vi "FindDevices.vi"(0 "Коммутатор Agilent 34980A":refnum<visa-resource-name>, 1 "Reset (True)":bool=TRUE, 5 "Мультиметр Agilent 34410A":refnum<visa-resource-name>, 7 "TP04300A":refnum<visa-resource-name>, 9 "Источник питания Agilent N6705A":refnum<visa-resource-name>) -> (4 "Статус коммутатора":bool, 6 "Статус вольтметра":bool, 8 "Статус камеры тепла/холода":bool, 10 "Статус источника питания":bool, 15 "error out":errorcluster)   [LabVIEW 2017]
uses:
  instr.lib/Temptronic TP04300/Temptronic TP04300.lvlib
  instr.lib/Agilent N6700 Series/Agilent N6700 Series.lvlib
panel:
  # "IN"
  # "OUT"
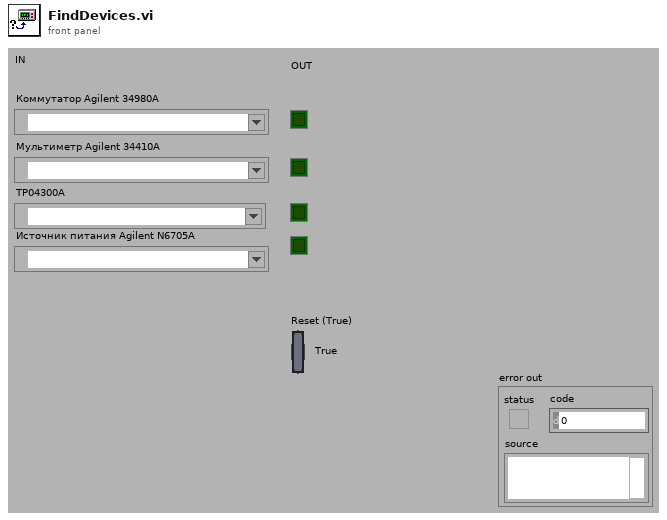
[diagram p1: front panel]
types:
  T1 = cluster{"Baud Rate":u32, "Parity":u16, "Data Bits":u16, "Stop Bits":u16, "Flow Control":u16}
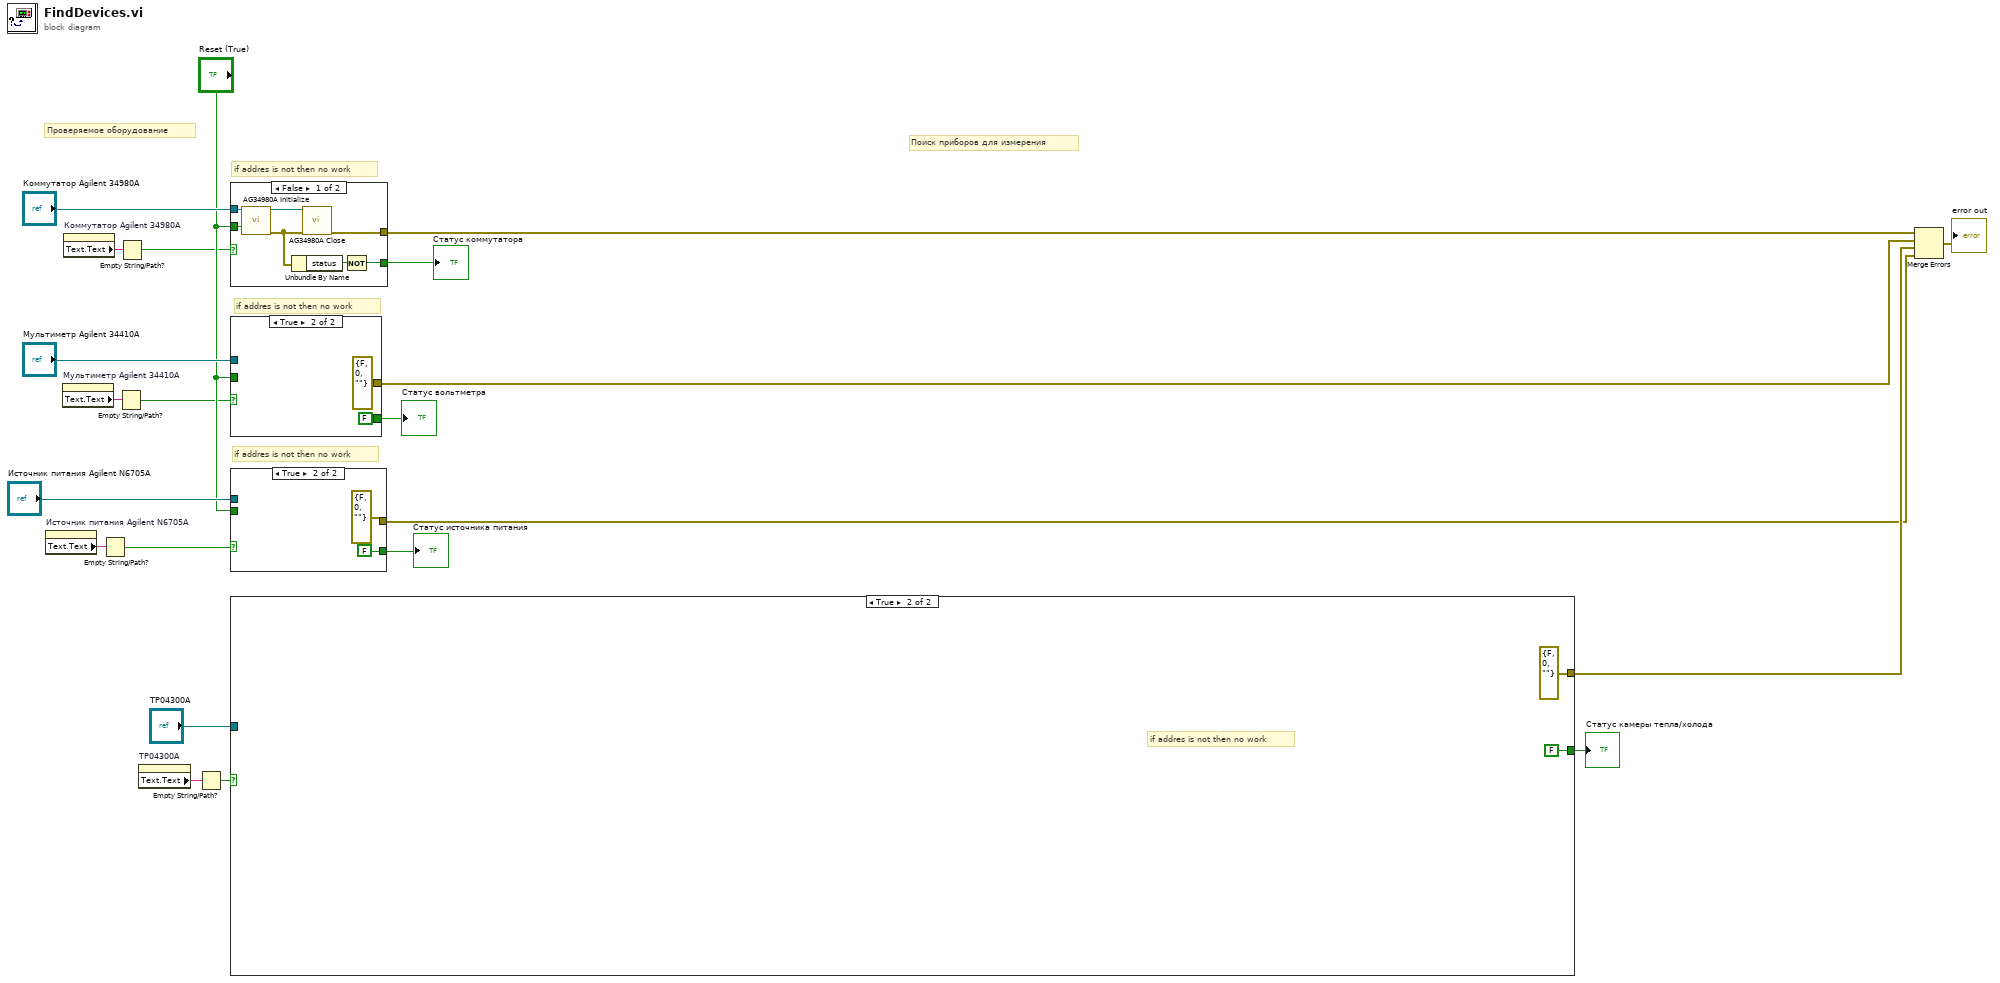
[diagram p0: block diagram]
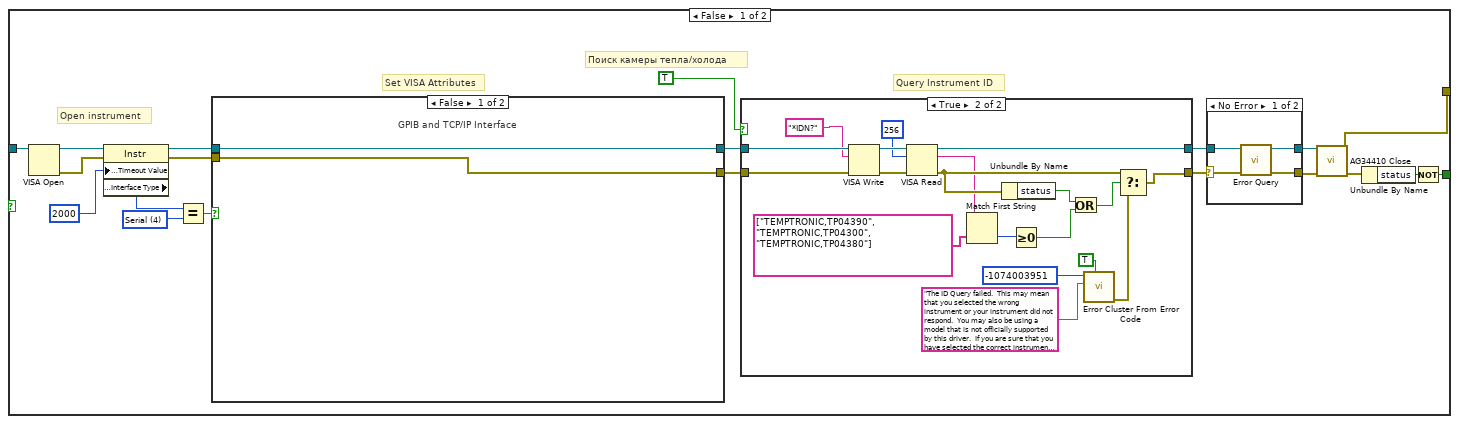
[diagram p2: hidden frame]
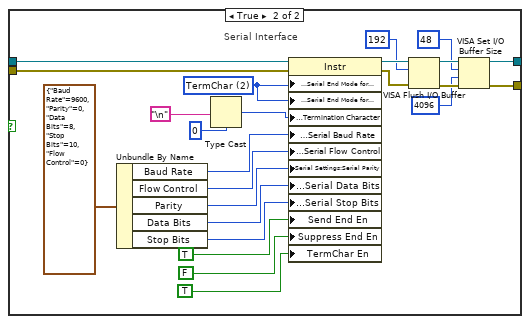
[diagram p3: hidden frame]
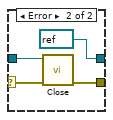
[diagram p4: hidden frame]
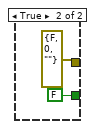
[diagram p6: hidden frame]
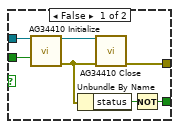
[diagram p7: hidden frame]
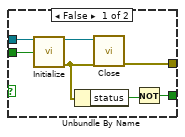
[diagram p8: hidden frame]
diagram:
  # "if addres is not then no work"
  # "if addres is not then no work"
  # "if addres is not then no work"
  # "if addres is not then no work"
  # "Проверяемое оборудование"
  # "Поиск приборов для измерения"
  n1 = property on="Источник питания Agilent N6705A" class="VISAName"() -> ("Text.Text"=w9:string)  [unwired: 2 in, 2 out]
  n2 = property on="Мультиметр Agilent 34410A" class="VISAName"() -> ("Text.Text"=w7:string)  [unwired: 2 in, 2 out]
  n3 = property on="Коммутатор Agilent 34980A" class="VISAName"() -> ("Text.Text"=w4:string)  [unwired: 2 in, 2 out]
  n4 = Empty String/Path?(string/path=w9) -> (empty?=w8:bool)
  n5 = Empty String/Path?(string/path=w7) -> (empty?=w6:bool)
  n6 = Empty String/Path?(string/path=w4) -> (empty?=w3:bool)
  n7 = property on="TP04300A" class="VISAName"() -> ("Text.Text"=w2:string)  [unwired: 2 in, 2 out]
  n8 = Empty String/Path?(string/path=w2) -> (empty?=w1:bool)
  n9 = case shown="False" w3 {
    tunnel: [w29 errorcluster {"status"=FALSE, "code"=0, "source"=""} ("error out")] -> w18
    tunnel: [w28 FALSE] -> w17
    tunnel: "Коммутатор Agilent 34980A" -> [w26 _]
    tunnel: "Reset (True)" -> [w23 _]
    frame False {
      n10 = call "AG34980A Initialize.vi"("VISA resource name"=w26, "Reset (True)"=w23) -> ("VISA session"=w25:refnum<visa-resource-name>, "error out"=w24:errorcluster)  [unwired: 12 in]
      n11 = Unbundle By Name(w24) -> ("status"=w27:bool)
      n12 = call "AG34980A Close.vi"("VISA resource name"=w25, "error in (no error)"=w24) -> ("error out"=w29:errorcluster)  [unwired: 13 in]
      n13 = Not(x=w27) -> (.not. x?=w28:bool)
    }
    frame True {
    }
  }
  "Статус коммутатора" <- w17
  n14 = case shown="True" w6 {
    tunnel: [w38 errorcluster {"status"=FALSE, "code"=0, "source"=""} ("error out")] -> w19
    tunnel: [w32 FALSE ("status")] -> w5
    tunnel: "Мультиметр Agilent 34410A" -> [w37 _]
    tunnel: "Reset (True)" -> [w34 _]
    frame False {
      n15 = call "AG34410 Initialize.vi"("VISA resource name"=w37, "Reset (True)"=w34) -> ("VISA resource name out"=w36:refnum<visa-resource-name>, "error out"=w35:errorcluster)  [unwired: 12 in]
      n16 = Unbundle By Name(w35) -> ("status"=w33:bool)
      n17 = call "AG34410 Close.vi"("VISA resource name"=w36, "error in (no error)"=w35) -> ("error out"=w38:errorcluster)  [unwired: 13 in]
      n18 = Not(x=w33) -> (.not. x?=w32:bool)
    }
    frame True {
    }
  }
  "Статус вольтметра" <- w5
  n19 = case shown="True" w8 {
    tunnel: "Источник питания Agilent N6705A" -> [w47 _]
    tunnel: "Reset (True)" -> [w46 _]
    tunnel: [w44 FALSE] -> w11
    tunnel: [w41 errorcluster {"status"=FALSE, "code"=0, "source"=""} ("error out")] -> w10
    frame False {
      n20 = call "Initialize.vi"("VISA resource name"=w47, "Reset? (T: Yes)"=w46) -> ("VISA resource name out"=w43:refnum<visa-resource-name>, "error out"=w42:errorcluster)  [unwired: 12 in]
      n21 = Unbundle By Name(w42) -> ("status"=w45:bool)
      n22 = call "Close.vi"("VISA resource name"=w43, "error in (no error)"=w42) -> ("error out"=w41:errorcluster)  [unwired: 13 in]
      n23 = Not(x=w45) -> (.not. x?=w44:bool)
    }
    frame True {
    }
  }
  "Статус источника питания" <- w11
  n24 = case shown="True" w1 {
    tunnel: [w68 errorcluster {"status"=FALSE, "code"=0, "source"=""} ("error out")] -> w22
    tunnel: [w52 FALSE] -> w21
    tunnel: "TP04300A" -> [w50 _]
    frame False {
      w60 = u16 4 items=["GPIB"=1, "VXI"=2, "GPIB-VXI"=3, "Serial"=4, "PXI"=5, "TCPIP"=6, "USB"=7] ("Interface Information:Interface Type")
      # "Поиск камеры тепла/холода"
      # "Set VISA Attributes"
      # "Query Instrument ID"
      # "Open instrument"
      n25 = VISA Open(VISA resource name=w50) -> (VISA resource name=w62:refnum<visa-resource-name>, error out=w61:errorcluster)  [unwired: 4 in]
      n26 = property class="Instr"(reference=w62, error in=w61, "General Settings:Timeout Value"=u32 2000) -> (reference out=w58:refnum<visa-resource-name>, error out=w59:errorcluster, "Interface Information:Interface Type"=w54:u16)
      n27 = Equal?(x=w54, y=w60) -> (x = y?=w63:bool)
      n28 = case shown="False" w63 {
        tunnel: [w69 w91] -> w56
        tunnel: [w70 w88] -> w57
        tunnel: w58 -> [w69 w93]
        tunnel: w59 -> [w70 w94]
        frame False {
          # "GPIB and TCP/IP Interface"
        }
        frame True {
          w71 = u16 2 items=["None", "Last Bit", "TermChar", "Break"] ("Serial Settings:End Mode for Writes")
          # "Serial Interface"
          n29 = Unbundle By Name(T1 {"Baud Rate"=9600, "Parity"=0, "Data Bits"=8, "Stop Bits"=10, "Flow Control"=0} ("Serial Configuration")) -> ("Baud Rate"=w81:u32, "Flow Control"=w77:u16, "Parity"=w79:u16, "Data Bits"=w80:u16, "Stop Bits"=w76:u16)
          n30 = Type Cast(type=u8 0, x="\n") -> (*(type *) &x=w82:u8)
          n31 = property class="Instr"(reference=w93, error in=w94, "Serial Settings:Serial End Mode for Reads"=w71, "Serial Settings:Serial End Mode for Writes"=w71, "Message Based Settings:Termination Character"=w82, "Serial Settings:Serial Baud Rate"=w81, "Serial Settings:Serial Flow Control"=w77, "Serial Settings:Serial Parity"=w79, "Serial Settings:Serial Data Bits"=w80, "Serial Settings:Serial Stop Bits"=w76, "Send End En"=TRUE, "Suppress End En"=FALSE, "TermChar En"=TRUE) -> (reference out=w87:refnum<visa-resource-name>, error out=w90:errorcluster)
          n32 = VISA Flush I/O Buffer(VISA resource name=w87, mask (16)=u16 192, error in (no error)=w90) -> (VISA resource name out=w92:refnum<visa-resource-name>, error out=w89:errorcluster)
          n33 = VISA Set I/O Buffer Size(VISA resource name=w92, mask (16)=u16 48, size (4096)=u32 4096 ("size (0)"), error in (no error)=w89) -> (VISA resource name out=w91:refnum<visa-resource-name>, error out=w88:errorcluster)
        }
      }
      n34 = case shown="True" TRUE ("ID Query (True)") {
        tunnel: [w103 w108] -> w65
        tunnel: [w104 w121] -> w64
        tunnel: w56 -> [w104 w122]
        tunnel: w57 -> [w103 w123]
        frame False {
        }
        frame True {
          n35 = VISA Write(VISA resource name=w122, write buffer="*IDN?", error in (no error)=w123) -> (VISA resource name out=w120:refnum<visa-resource-name>, error out=w119:errorcluster)  [unwired: 1 out]
          n36 = VISA Read(VISA resource name=w120, byte count=u32 256, error in (no error)=w119) -> (VISA resource name out=w121:refnum<visa-resource-name>, read buffer=w107:string, error out=w110:errorcluster)  [unwired: 1 out]
          n37 = Match First String(2:string[] ["TEMPTRONIC,TP04390", "TEMPTRONIC,TP04300", "TEMPTRONIC,TP04380"] ("string array"), 3:w107) -> (0:w105:i32)  [unwired: 1 out]
          n38 = Unbundle By Name(w110) -> ("status"=w115:bool)
          n39 = Greater Or Equal To 0?(x=w105) -> (x >= 0?=w116:bool)
          n40 = Or(x=w115, y=w116) -> (x .or. y?=w109:bool)
          n41 = call <vilib>:"Error Cluster From Error Code.vi"("show call chain? (False)"=TRUE, "error message (\"\")"="The ID Query failed.  This may mean that you selected the wrong instrument or your instrument did not respond.  You may also be using a model that is not officially supported by this driver.  If you are sure that you have selected the correct instrument and it is responding, try disabling the ID Query." ("Source (VI Name)"), "error code (0)"=-1074003951 ("Code")) -> ("error out"=w111:errorcluster)  [unwired: 6 in]
          n42 = Select(t=w110, s=w109, f=w111) -> (s? t:f=w108:errorcluster)
        }
      }
      n43 = case shown="No Error" w65 {
        selector: w65 -> [w96 w100]
        tunnel: w64 -> [w95 w101]
        tunnel: [w98 refnum<visa-resource-name> refnum ("VISA resource name out")] -> w66
        tunnel: [w97 w102] -> w67
        frame No Error {
          n44 = call "Error Query.vi"("error in (no error)"=w96, "VISA resource name"=w95) -> ("error out"=w97:errorcluster, "VISA resource name out"=w98:refnum<visa-resource-name>)  [unwired: 6 in, 2 out]
        }
        frame Error {
          n45 = call "Close.vi"("error in (no error)"=w100, "VISA resource name"=w101) -> ("error out"=w102:errorcluster)  [unwired: 9 in]
        }
      }
      n46 = call "AG34410 Close.vi"("VISA resource name"=w66, "error in (no error)"=w67) -> ("error out"=w68:errorcluster)  [unwired: 13 in]
      n47 = Unbundle By Name(w68) -> ("status"=w51:bool)
      n48 = Not(x=w51) -> (.not. x?=w52:bool)
    }
    frame True {
    }
  }
  "Статус камеры тепла/холода" <- w21
  n49 = Merge Errors(w18, w19, w22, w10) -> (→"error out":errorcluster)
